vi "动力和环境监控系统状态详情.vi"() -> ()   [LabVIEW 2016, in "环境动力监测库.lvlib"]
uses:
  <vilib>/Utility/miscctls.llb/LVRowAndColumnTypeDef.ctl
  <vilib>/Utility/config.llb/NI_LVConfig.lvlib
  <vilib>/ptbypt/NI_PtbyPt.lvlib
panel:
  out "网络状态":bool
  in  "监测设备更新":bool
  in  "设备列表":i32(listbox)
  in  "add":bool
  out "设备当前时间:":timestamp format="%<%Y/%m/%d %H:%M:%S>T"
  out "当前传感器数量:":i32
  in  "设备":T1(ring)
  # "系统当前状态"
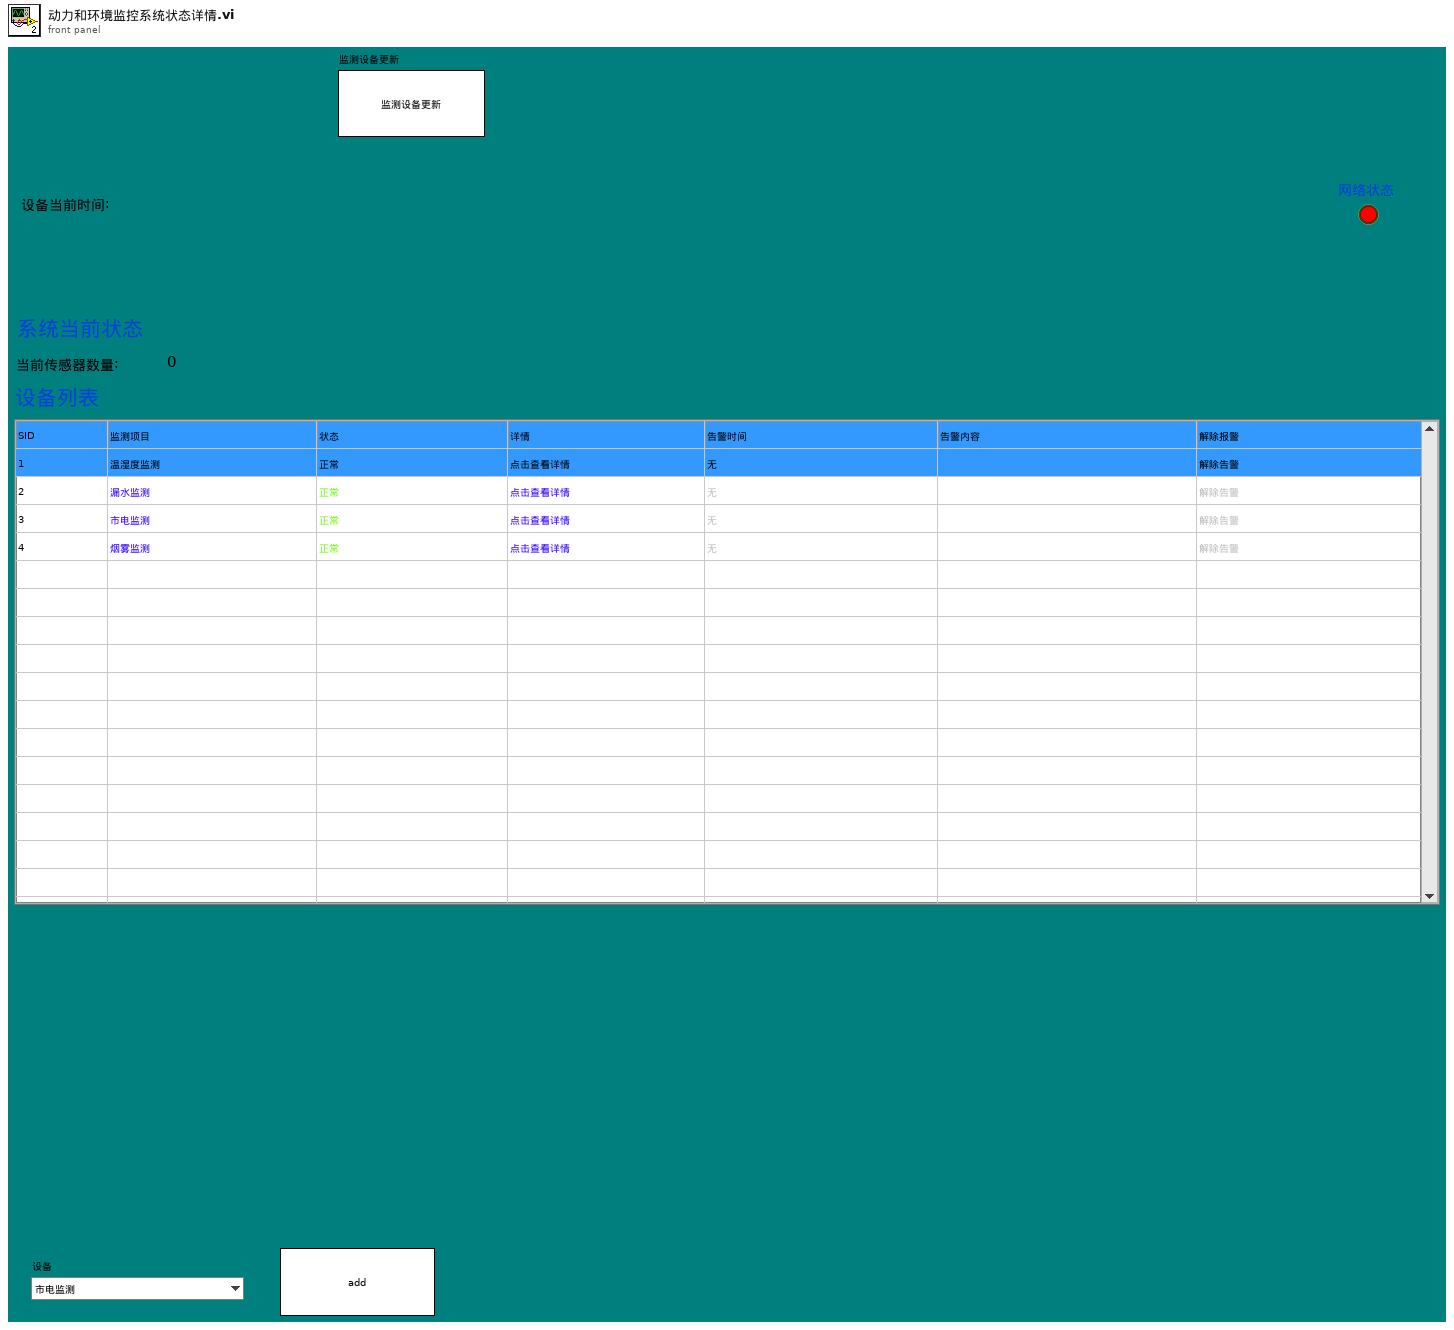
[diagram p1: front panel]
types:
  T1 = enum16{"市电监测", "UPS监测", "用水量监测", "空调监测", "烟雾监测", "温度湿度", "振动监测", "红外入侵监测", "漏水监测", "门禁开关监测", "视频监测"}
  T2 = typedef "NI_LVConfig.lvlib/Config Data RefNum.ctl" = refnum<k1>
  T3 = cluster{"市电监测":bool, "用水量监测":bool, "烟雾监测":bool, "温度湿度":bool, "振动监测":bool, "红外入侵监测":bool, "漏水监测":bool, "门禁开关监测":bool, "门禁开关监测2":bool, "视频监测":bool, "UPS监测":bool, "空调监测":bool, "冰箱监测":bool, "排气扇监测":bool, "蓄电池监测":bool, "蓄电池监测2":bool, "GPS监测":bool, "北斗监测":bool, "气象监测":bool}
  T4 = enum32{"Invalid", "Standard", "Closed", "Hidden", "Minimized", "Maximized"}
  T5 = cluster{"漏水监测输出":cluster{"漏水监测告警":bool, "告警内容":string}, "门禁监测输出":cluster{"门禁监测告警":bool, "告警内容":string}, "门禁监测输出2":cluster{"门禁监测告警":bool, "告警内容":string}, "温湿度监测输出":cluster{"温湿度监测告警":bool, "告警内容":string}, "烟雾监测输出":cluster{"烟雾监测告警":bool, "告警内容":string}, "空调监测输出":cluster{"空调监测告警":bool, "告警内容":string}, "自动重合闸输出":cluster{"自动重合闸告警":bool, "告警内容":string}, "红外入侵输出":cluster{"红外入侵告警":bool, "告警内容":string}, "振动输出":cluster{"振动告警":bool, "告警内容":string}, "UPS输出":cluster{"UPS告警":bool, "告警内容":string}, "蓄电池输出":cluster{"蓄电池告警":bool, "告警内容":string}, "蓄电池输出2":cluster{"蓄电池告警":bool, "告警内容":string}, "GPS输出":cluster{"定位告警":bool, "告警内容":string}, "北斗输出":cluster{"定位告警":bool, "告警内容":string}, "气象输出":cluster{"气象告警":bool, "告警内容":string}}
  T6 = typedef "LVRowAndColumnTypeDef.ctl" = cluster{"Row":i32, "Column":i32}
  T7 = typedef "LVPoint32TypeDef.ctl" = cluster{"Horizontal":i32, "Vertical":i32}
  T8 = enum32{"Bad", "Idle", "Run top level", "Running"}
  T9 = cluster{"AD0":dbl, "AD1":dbl, "AD1":dbl, "AD3":dbl, "AD4":dbl, "AD5":dbl, "AD6":dbl, "AD7":dbl}
  T10 = cluster{"X0":dbl, "X1":dbl, "Y0":dbl, "Y1":dbl}[]
  T11 = cluster{"AD0":dbl, "AD1":dbl, "AD2":dbl, "AD3":dbl, "AD4":dbl, "AD5":dbl, "AD6":dbl, "AD7":dbl}
  T12 = cluster{"温湿度":cluster{"状态":bool, "温度:":sgl, "湿度:":sgl, "详情  ":bool}, "空调":cluster{"状态":bool, "机柜温度:":sgl, "压缩机:":enum16{"停止", "运行"}, "电加热:":enum16{"停止", "运行"}, "详情  ":bool}, "排气扇":cluster{"排气扇:":enum16{"关闭", "打开"}, "详情  ":bool}, "冰箱":cluster{"冰箱:":enum16{"关闭", "打开"}, "详情  ":bool}}
  T13 = cluster{"市电":cluster{"状态":bool, "电压:":u16, "电流：":dbl, "详情  ":bool}, "UPS":cluster{"状态":bool, "输入电压:":sgl, "输出电压:":sgl, "电池电量:":u8, "电量":u16, "详情  ":bool}, "蓄电池12V":cluster{"状态":bool, "电压:":sgl, "电流:":sgl, "电池电量:":u8, "电量":u16, "详情  ":bool}, "蓄电池24V":cluster{"状态":bool, "电压:":sgl, "电流:":sgl, "电池电量:":u8, "电量":u16, "详情  ":bool}}
  T14 = cluster{"传感器":cluster{"红外监测":cluster{"红外监测":bool, "红外入侵监测":bool}, "振动监测":cluster{"振动监测":bool, "振动监测 2":bool}, "烟雾监测":cluster{"烟雾监测":bool, "烟雾监测 2":bool}, "门禁监测":cluster{"门禁监测":bool, "门禁开关监测":bool}, "门禁2监测":cluster{"门禁监测2":bool, "门禁开关监测2":bool}, "水浸监测":cluster{"水浸监测":bool, "漏水详情":bool}}, "气象仪":cluster{"气温: ":sgl, "气压: ":sgl, "风速:":sgl, "风向:":sgl, "气象仪经度: ":sgl, "气象仪纬度: ":sgl, "详情  ":bool}}
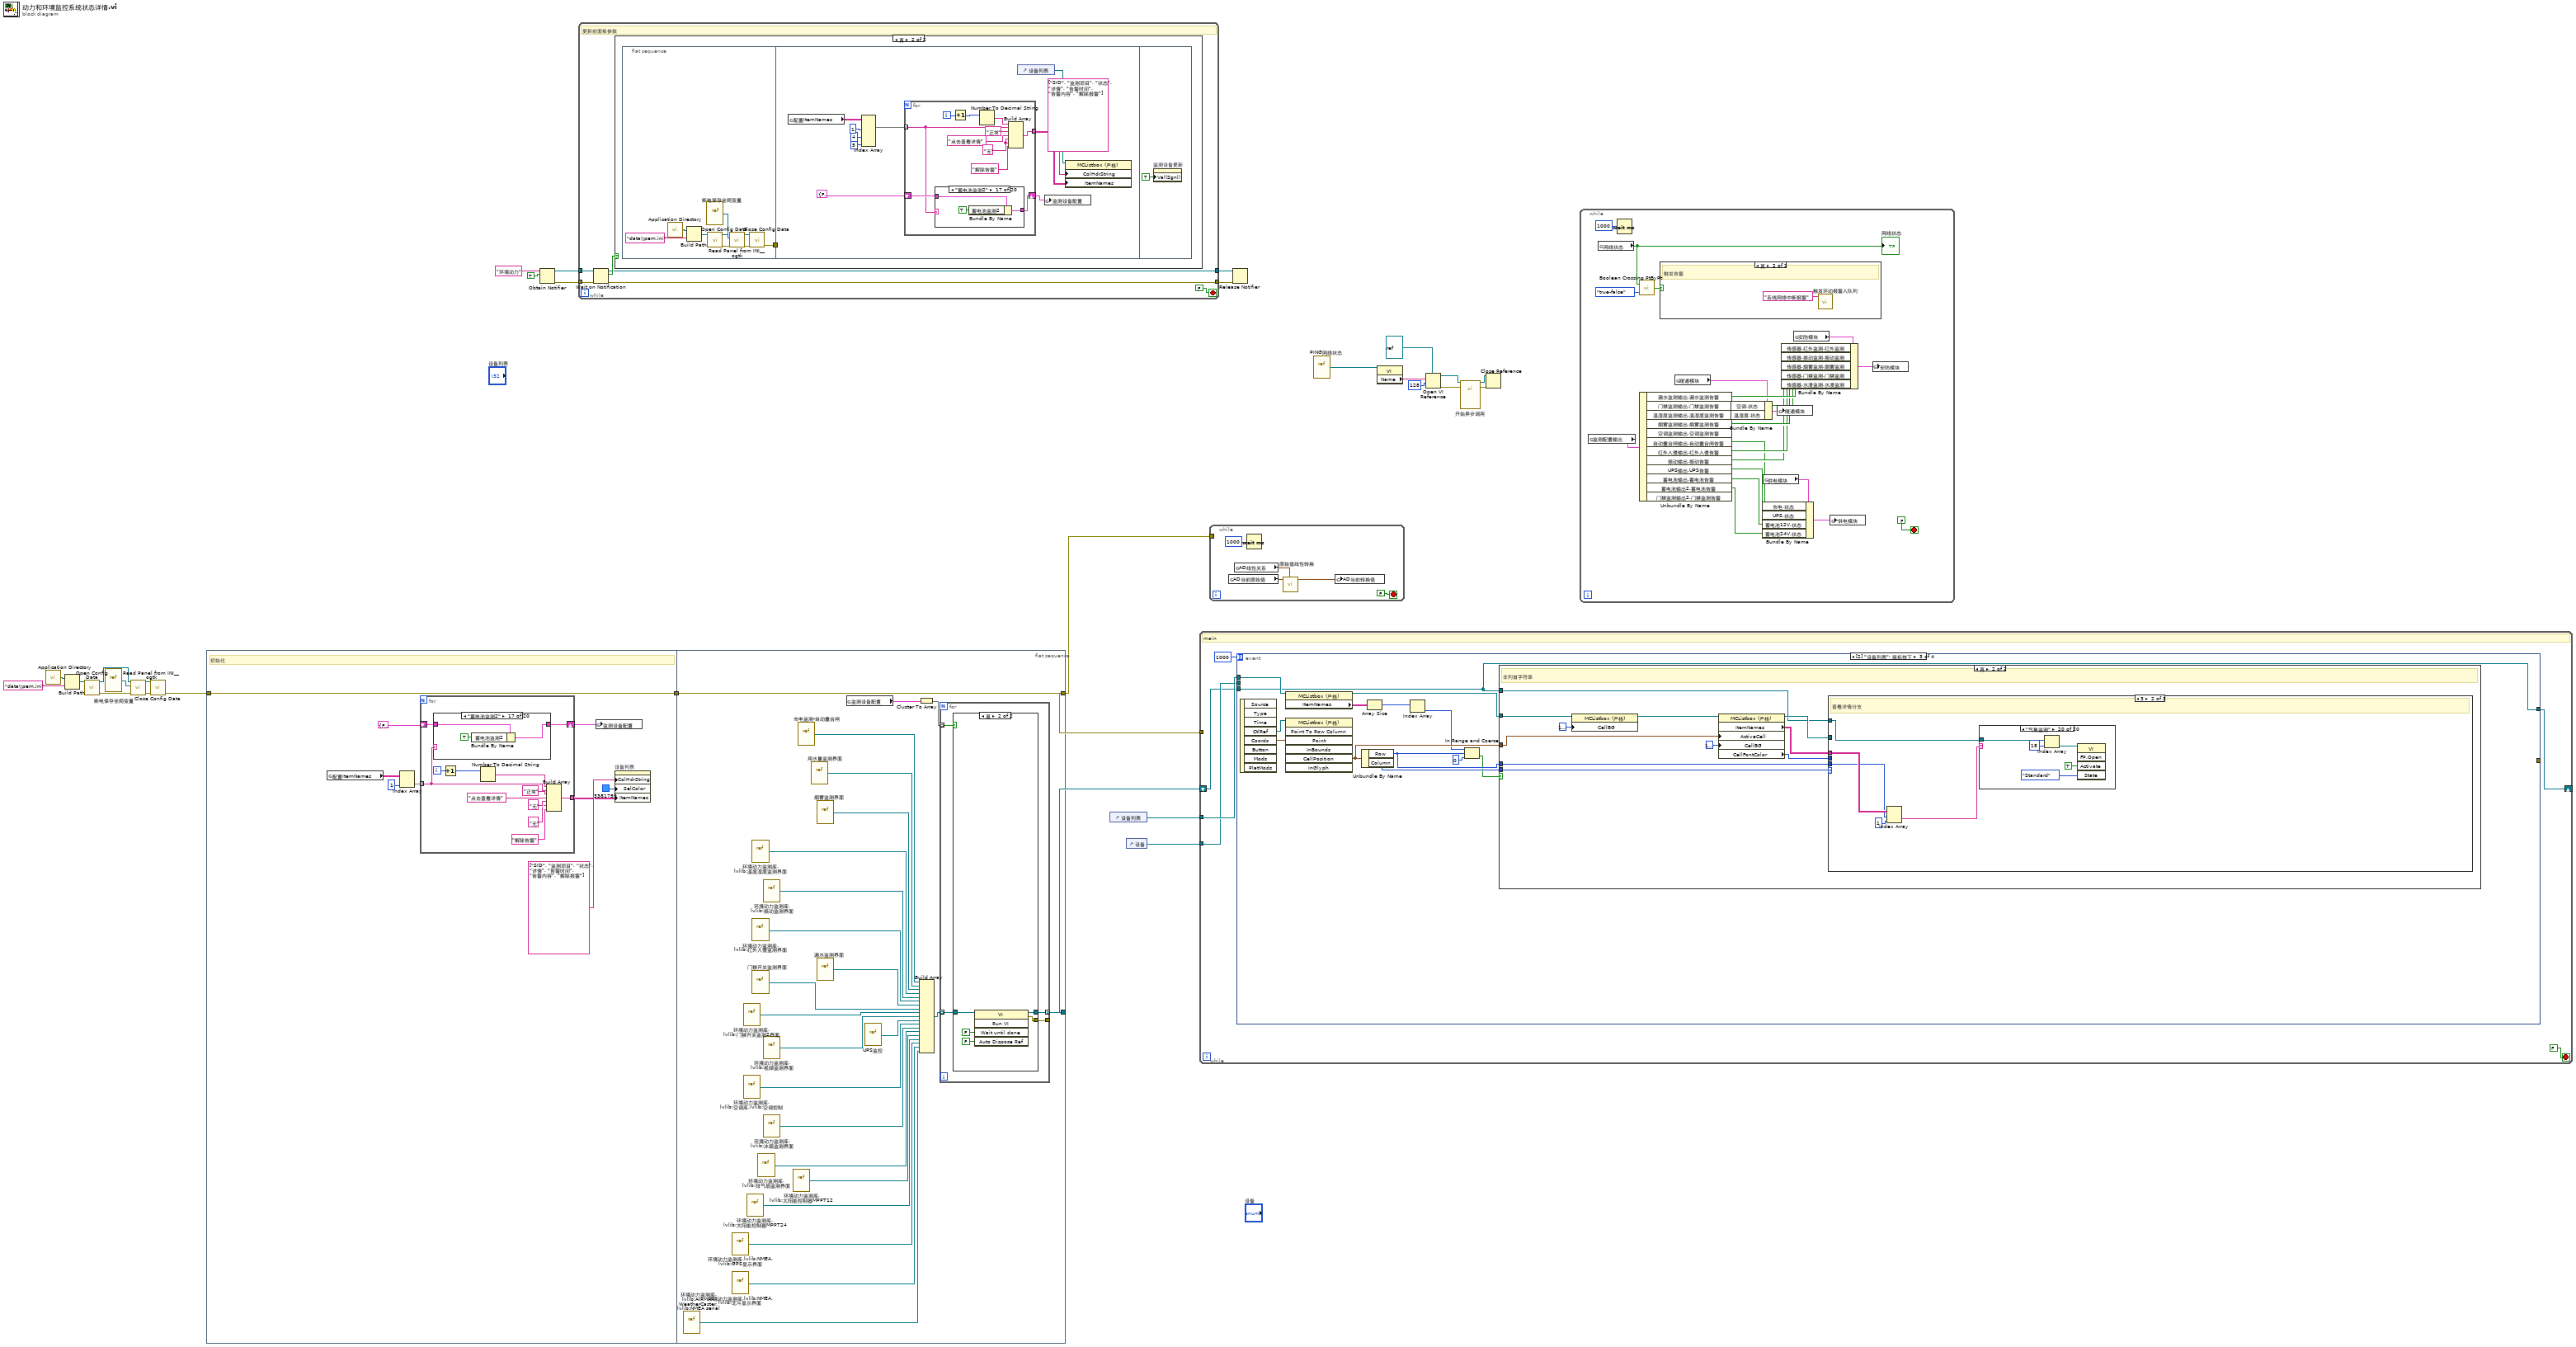
[diagram p0: block diagram]
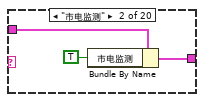
[diagram p5: hidden frame]
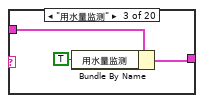
[diagram p6: hidden frame]
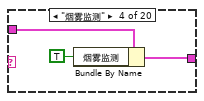
[diagram p7: hidden frame]
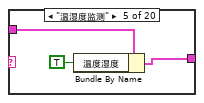
[diagram p8: hidden frame]
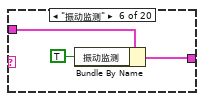
[diagram p9: hidden frame]
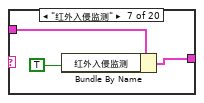
[diagram p10: hidden frame]
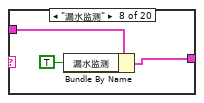
[diagram p11: hidden frame]
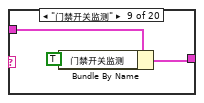
[diagram p12: hidden frame]
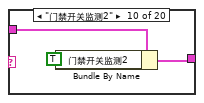
[diagram p13: hidden frame]
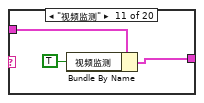
[diagram p14: hidden frame]
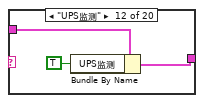
[diagram p15: hidden frame]
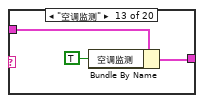
[diagram p16: hidden frame]
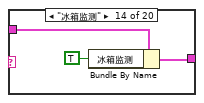
[diagram p17: hidden frame]
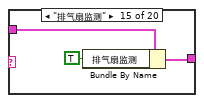
[diagram p18: hidden frame]
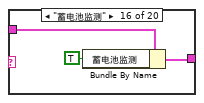
[diagram p19: hidden frame]
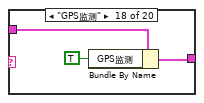
[diagram p20: hidden frame]
diagram:
  n1 = call <vilib>:"Application Directory.vi"() -> ("Application Directory"=w26:path)
  n2 = Build Path(base path=w26, name or relative path="data\\pem.ini" ("名称或相对路径")) -> (appended path=w24:path)
  n3 = call <vilib>:"Open Config Data.vi"("configuration file path"=w24) -> ("error out"=w20:errorcluster, "refnum"=w23:T2)  [unwired: 8 in, 1 out]
  n4 = vi-ref "断电保存全局变量.vi"() -> (w22:refnum<vi>)
  n5 = call <userlib>:"Read Panel from INI__ogtk.vi"("error in (no error)"=w20, "VI ref"=w22, "refnum"=w23) -> ("error out"=w19:errorcluster, "refnum out"=w21:T2)  [unwired: 7 in]
  n6 = call <vilib>:"Close Config Data.vi"("error in (no error)"=w19, "refnum"=w21) -> ("error out"=w18:errorcluster)  [unwired: 8 in, 1 out]
  n7 = flat-sequence {
    tunnel: [w31] -> w13
    tunnel: w18 -> [w31]
    tunnel: [w131] -> w1
    tunnel: w13 -> [w131]
    tunnel: [w118] -> w12
    frame #0 {
      # "初始化"
      n8 = global read "断电保存全局变量.vi" "配置ItemNames"() -> (w35:string[][])
      n9 = Index Array(array=w35, index (col)=1 ("禁用的索引 (列)")) -> (element=w33:string[])  [unwired: 1 in]
      n10 = for {
        tunnel: w33 -> [w40] mode=indexing
        tunnel: [w44] -> w32 mode=indexing
        shift-right: [w38] -> w29
        shift-left: T3 {"市电监测"=FALSE, "用水量监测"=FALSE, "烟雾监测"=FALSE, "温度湿度"=FALSE, "振动监测"=FALSE, "红外入侵监测"=FALSE, "漏水监测"=FALSE, "门禁开关监测"=FALSE, "门禁开关监测2"=FALSE, "视频监测"=FALSE, "UPS监测"=FALSE, "空调监测"=FALSE, "冰箱监测"=FALSE, "排气扇监测"=FALSE, "蓄电池监测"=FALSE, "蓄电池监测2"=FALSE, "GPS监测"=FALSE, "北斗监测"=FALSE, "气象监测"=FALSE} ("监测设备配置") -> [w39]
        i -> [w49]
        n11 = case shown="\"蓄电池监测2\"" w40 {
          tunnel: w39 -> [w50 w53 w55 w58 w61 w64 w67 w70 w73 w76 w79 w82 w85 w88 w91 w94 w97 w100 w103 w106]
          tunnel: [w50 w51 w54 w57 w60 w63 w66 w69 w72 w75 w78 w81 w84 w87 w90 w93 w96 w99 w102 w105] -> w38
          frame "假", Default {
          }
          frame "市电监测" {
            n12 = Bundle By Name(cluster=w53, "市电监测"=TRUE) -> (w51:T3)
          }
          frame "用水量监测" {
            n13 = Bundle By Name(cluster=w55, "用水量监测"=TRUE ("市电监测")) -> (w54:T3)
          }
          frame "烟雾监测" {
            n14 = Bundle By Name(cluster=w58, "烟雾监测"=TRUE ("市电监测")) -> (w57:T3)
          }
          frame "温湿度监测" {
            n15 = Bundle By Name(cluster=w61, "温度湿度"=TRUE ("市电监测")) -> (w60:T3)
          }
          frame "振动监测" {
            n16 = Bundle By Name(cluster=w64, "振动监测"=TRUE ("市电监测")) -> (w63:T3)
          }
          frame "红外入侵监测" {
            n17 = Bundle By Name(cluster=w67, "红外入侵监测"=TRUE ("市电监测")) -> (w66:T3)
          }
          frame "漏水监测" {
            n18 = Bundle By Name(cluster=w70, "漏水监测"=TRUE ("市电监测")) -> (w69:T3)
          }
          frame "门禁开关监测" {
            n19 = Bundle By Name(cluster=w73, "门禁开关监测"=TRUE ("市电监测")) -> (w72:T3)
          }
          frame "门禁开关监测2" {
            n20 = Bundle By Name(cluster=w76, "门禁开关监测2"=TRUE ("市电监测")) -> (w75:T3)
          }
          frame "视频监测" {
            n21 = Bundle By Name(cluster=w79, "视频监测"=TRUE ("市电监测")) -> (w78:T3)
          }
          frame "UPS监测" {
            n22 = Bundle By Name(cluster=w82, "UPS监测"=TRUE ("市电监测")) -> (w81:T3)
          }
          frame "空调监测" {
            n23 = Bundle By Name(cluster=w85, "空调监测"=TRUE ("市电监测")) -> (w84:T3)
          }
          frame "冰箱监测" {
            n24 = Bundle By Name(cluster=w88, "冰箱监测"=TRUE ("市电监测")) -> (w87:T3)
          }
          frame "排气扇监测" {
            n25 = Bundle By Name(cluster=w91, "排气扇监测"=TRUE ("市电监测")) -> (w90:T3)
          }
          frame "蓄电池监测" {
            n26 = Bundle By Name(cluster=w94, "蓄电池监测"=TRUE ("市电监测")) -> (w93:T3)
          }
          frame "蓄电池监测2" {
            n27 = Bundle By Name(cluster=w97, "蓄电池监测2"=TRUE ("市电监测")) -> (w96:T3)
          }
          frame "GPS监测" {
            n28 = Bundle By Name(cluster=w100, "GPS监测"=TRUE ("市电监测")) -> (w99:T3)
          }
          frame "北斗监测" {
            n29 = Bundle By Name(cluster=w103, "北斗监测"=TRUE ("市电监测")) -> (w102:T3)
          }
          frame "气象监测" {
            n30 = Bundle By Name(cluster=w106, "气象监测"=TRUE ("市电监测")) -> (w105:T3)
          }
        }
        n31 = Increment(x=w49) -> (x+1=w48:i32)
        n32 = Number To Decimal String(number=w48) -> (decimal integer string=w47:string)  [unwired: 1 in]
        n33 = Build Array(w47, w40, "正常" ("元素"), "点击查看详情" ("元素"), "无" ("元素"), "无" ("元素"), "解除告警" ("元素")) -> (w44:string[])
      }
      n34 = global write "断电保存全局变量.vi" "监测设备配置"(w29) -> ()
      n35 = property on="设备列表" class="MCListbox (严格)"("ColHdrString"=string[] ["SID", "监测项目", "状态", "详情", "告警时间", "告警内容", "解除报警"] ("列首字符串[]"), "SelColor"=u32 3381759, "ItemNames"=w32) -> ()  [unwired: 2 in, 2 out]
    }
    frame #1 {
      n36 = vi-ref "环境动力监测库.lvlib:AIRMAR WeatherCaster.lvlib:NMEA serial.vi"() -> (w114:refnum<vi>)
      n37 = vi-ref "环境动力监测库.lvlib:NMEA.lvlib:GPS显示界面.vi"() -> (w115:refnum<vi>)
      n38 = vi-ref "环境动力监测库.lvlib:NMEA.lvlib:北斗显示界面.vi"() -> (w113:refnum<vi>)
      n39 = vi-ref "环境动力监测库.lvlib:门禁开关监测2界面.vi"() -> (w109:refnum<vi>)
      n40 = vi-ref "环境动力监测库.lvlib:空调库.lvlib:空调控制.vi"() -> (w129:refnum<vi>)
      n41 = vi-ref "环境动力监测库.lvlib:太阳能控制器MPPT24.vi"() -> (w111:refnum<vi>)
      n42 = vi-ref "环境动力监测库.lvlib:温度湿度监测界面.vi"() -> (w123:refnum<vi>)
      n43 = vi-ref "环境动力监测库.lvlib:红外入侵监测界面.vi"() -> (w125:refnum<vi>)
      n44 = vi-ref "门禁开关监测界面.vi"() -> (w108:refnum<vi>)
      n45 = vi-ref "环境动力监测库.lvlib:排气扇监测界面.vi"() -> (w117:refnum<vi>)
      n46 = vi-ref "环境动力监测库.lvlib:振动监测界面.vi"() -> (w124:refnum<vi>)
      n47 = vi-ref "环境动力监测库.lvlib:视频监测界面.vi"() -> (w127:refnum<vi>)
      n48 = vi-ref "环境动力监测库.lvlib:冰箱监测界面.vi"() -> (w116:refnum<vi>)
      n49 = vi-ref "环境动力监测库.lvlib:太阳能控制器MPPT12.vi"() -> (w110:refnum<vi>)
      n50 = vi-ref "市电监测-自动重合闸.vi"() -> (w120:refnum<vi>)
      n51 = vi-ref "用水量监测界面.vi"() -> (w121:refnum<vi>)
      n52 = vi-ref "烟雾监测界面.vi"() -> (w122:refnum<vi>)
      n53 = vi-ref "漏水监测界面.vi"() -> (w126:refnum<vi>)
      n54 = global read "断电保存全局变量.vi" "监测设备配置"() -> (w112:T3)
      n55 = vi-ref "UPS监控.vi"() -> (w128:refnum<vi>)
      n56 = Cluster To Array(cluster=w112) -> (array=w130:bool[])
      n57 = Build Array(w120, w121, w122, w123, w124, w125, w126, w108, w109, w127, w128, w129, w116, w117, w110, w111, w115, w113, w114) -> (w119:refnum<vi>[])
      n58 = for {
        tunnel: w119 -> [w135] mode=indexing
        tunnel: [w134] -> w118 mode=indexing
        tunnel: w130 -> [w133] mode=indexing
        tunnel: [w132] -> _
        n59 = case shown="真" w133 {
          tunnel: w135 -> [w136 w139]
          tunnel: [w136 w138] -> w134
          tunnel: [_ w137] -> w132
          frame False {
          }
          frame True {
            n60 = invoke class="VI" method="Run VI"(reference=w139, "Wait until done"=FALSE ("结束前等待"), "Auto Dispose Ref"=FALSE ("自动销毁引用")) -> (reference out=w138:refnum<vi>, error out=w137:errorcluster)  [unwired: 2 in, 3 out]
          }
        }
      }
    }
  }
  n61 = Obtain Notifier(name (unnamed)="环境动力" ("名称（未命名）"), notification data type=TRUE) -> (notifier out=w3:refnum<notifier>, error out=w2:errorcluster)  [unwired: 2 in, 1 out]
  n62 = while {
    tunnel: w3 -> [w147]
    tunnel: w2 -> [w146]
    tunnel: [w143] -> w15
    tunnel: [w142] -> w14
    stop <- FALSE stop-if-true
    # "更新前面板参数"
    n63 = Wait on Notification(notifier=w147, error in (no error)=w146) -> (notifier out=w143:refnum<notifier>, notification=w145:bool, error out=w142:errorcluster)  [unwired: 2 in, 1 out]
    n64 = case shown="真" w145 {
      frame False {
      }
      frame True {
        n65 = flat-sequence {
          tunnel: [w149] -> w148
          tunnel: w148 -> [_]
          frame #0 {
            n66 = call <vilib>:"Application Directory.vi"() -> ("Application Directory"=w150:path)
            n67 = Build Path(base path=w150, name or relative path="data\\pem.ini" ("名称或相对路径")) -> (appended path=w152:path)
            n68 = vi-ref "断电保存全局变量.vi"() -> (w154:refnum<vi>)
            n69 = call <vilib>:"Open Config Data.vi"("configuration file path"=w152) -> ("error out"=w156:errorcluster, "refnum"=w153:T2)  [unwired: 8 in, 1 out]
            n70 = call <userlib>:"Read Panel from INI__ogtk.vi"("error in (no error)"=w156, "VI ref"=w154, "refnum"=w153) -> ("error out"=w157:errorcluster, "refnum out"=w155:T2)  [unwired: 7 in]
            n71 = call <vilib>:"Close Config Data.vi"("error in (no error)"=w157, "refnum"=w155) -> ("error out"=w149:errorcluster)  [unwired: 8 in, 1 out]
          }
          frame #1 {
            n72 = global read "断电保存全局变量.vi" "配置ItemNames"() -> (w162:string[][])
            n73 = Index Array(array=w162, index (col) #1=1 ("禁用的索引 (列)"), index (col) #2=4 ("索引 (列)"), index (col) #3=5 ("索引 (列)")) -> (element #1=w164:string[])  [unwired: 3 in, 2 out]
            n74 = for {
              tunnel: w164 -> [w170] mode=indexing
              tunnel: [w173] -> w167 mode=indexing
              shift-right: [w171] -> w161
              shift-left: T3 {"市电监测"=FALSE, "用水量监测"=FALSE, "烟雾监测"=FALSE, "温度湿度"=FALSE, "振动监测"=FALSE, "红外入侵监测"=FALSE, "漏水监测"=FALSE, "门禁开关监测"=FALSE, "门禁开关监测2"=FALSE, "视频监测"=FALSE, "UPS监测"=FALSE, "空调监测"=FALSE, "冰箱监测"=FALSE, "排气扇监测"=FALSE, "蓄电池监测"=FALSE, "蓄电池监测2"=FALSE, "GPS监测"=FALSE, "北斗监测"=FALSE, "气象监测"=FALSE} ("监测设备配置") -> [w172]
              i -> [w178]
              w168 = "无" ("元素")
              n75 = case shown="\"蓄电池监测2\"" w170 {
                tunnel: w172 -> [w179 w182 w184 w187 w190 w193 w196 w199 w202 w205 w208 w211 w214 w217 w220 w223 w226 w229 w232 w235]
                tunnel: [w179 w180 w183 w186 w189 w192 w195 w198 w201 w204 w207 w210 w213 w216 w219 w222 w225 w228 w231 w234] -> w171
                frame "假", Default {
                }
                frame "市电监测" {
                  n76 = Bundle By Name(cluster=w182, "市电监测"=TRUE) -> (w180:T3)
                }
                frame "用水量监测" {
                  n77 = Bundle By Name(cluster=w184, "用水量监测"=TRUE ("市电监测")) -> (w183:T3)
                }
                frame "烟雾监测" {
                  n78 = Bundle By Name(cluster=w187, "烟雾监测"=TRUE ("市电监测")) -> (w186:T3)
                }
                frame "温湿度监测" {
                  n79 = Bundle By Name(cluster=w190, "温度湿度"=TRUE ("市电监测")) -> (w189:T3)
                }
                frame "振动监测" {
                  n80 = Bundle By Name(cluster=w193, "振动监测"=TRUE ("市电监测")) -> (w192:T3)
                }
                frame "红外入侵监测" {
                  n81 = Bundle By Name(cluster=w196, "红外入侵监测"=TRUE ("市电监测")) -> (w195:T3)
                }
                frame "漏水监测" {
                  n82 = Bundle By Name(cluster=w199, "漏水监测"=TRUE ("市电监测")) -> (w198:T3)
                }
                frame "门禁开关监测" {
                  n83 = Bundle By Name(cluster=w202, "门禁开关监测"=TRUE ("市电监测")) -> (w201:T3)
                }
                frame "门禁开关监测2" {
                  n84 = Bundle By Name(cluster=w205, "门禁开关监测2"=TRUE ("市电监测")) -> (w204:T3)
                }
                frame "视频监测" {
                  n85 = Bundle By Name(cluster=w208, "视频监测"=TRUE ("市电监测")) -> (w207:T3)
                }
                frame "UPS监测" {
                  n86 = Bundle By Name(cluster=w211, "UPS监测"=TRUE ("市电监测")) -> (w210:T3)
                }
                frame "空调监测" {
                  n87 = Bundle By Name(cluster=w214, "空调监测"=TRUE ("市电监测")) -> (w213:T3)
                }
                frame "冰箱监测" {
                  n88 = Bundle By Name(cluster=w217, "冰箱监测"=TRUE ("市电监测")) -> (w216:T3)
                }
                frame "排气扇监测" {
                  n89 = Bundle By Name(cluster=w220, "排气扇监测"=TRUE ("市电监测")) -> (w219:T3)
                }
                frame "蓄电池监测" {
                  n90 = Bundle By Name(cluster=w223, "蓄电池监测"=TRUE ("市电监测")) -> (w222:T3)
                }
                frame "蓄电池监测2" {
                  n91 = Bundle By Name(cluster=w226, "蓄电池监测2"=TRUE ("市电监测")) -> (w225:T3)
                }
                frame "GPS监测" {
                  n92 = Bundle By Name(cluster=w229, "GPS监测"=TRUE ("市电监测")) -> (w228:T3)
                }
                frame "北斗监测" {
                  n93 = Bundle By Name(cluster=w232, "北斗监测"=TRUE ("市电监测")) -> (w231:T3)
                }
                frame "气象监测" {
                  n94 = Bundle By Name(cluster=w235, "气象监测"=TRUE ("市电监测")) -> (w234:T3)
                }
              }
              n95 = Increment(x=w178) -> (x+1=w177:i32)
              n96 = Number To Decimal String(number=w177) -> (decimal integer string=w176:string)  [unwired: 1 in]
              n97 = Build Array(w176, w170, "正常" ("元素"), "点击查看详情" ("元素"), w168, w168, "解除告警" ("元素")) -> (w173:string[])
            }
            n98 = control-ref of="设备列表"() -> (w165:refnum<vi>)
            n99 = global write "断电保存全局变量.vi" "监测设备配置"(w161) -> ()
            n100 = property class="MCListbox (严格)"(reference=w165, "ColHdrString"=string[] ["SID", "监测项目", "状态", "详情", "告警时间", "告警内容", "解除报警"] ("列首字符串[]"), "ItemNames"=w167) -> ()  [unwired: 1 in, 2 out]
          }
          frame #2 {
            n101 = property on="监测设备更新" class="Bool (严格)"("Val(Sgnl)"=TRUE ("值(信号)")) -> ()  [unwired: 2 in, 2 out]
          }
        }
      }
    }
  }
  n102 = control-ref of="设备列表"() -> (w28:refnum<vi>)
  n103 = control-ref of="设备"() -> (w27:refnum<vi>)
  n104 = while {
    tunnel: w28 -> [w242]
    tunnel: w27 -> [w241]
    tunnel: w1 -> [_]
    shift-right: [w238] -> _
    shift-left: w12 -> [w239]
    stop <- FALSE stop-if-true
    # "main"
    n105 = event shown="[2] \"设备列表\": 鼠标按下" {
      selector: _ -> [_ _ _ _]
      dyn-events: _ -> [_ _ _ _]
      timeout: 1000 -> [_ _ _ _]
      tunnel: w242 -> [_ w412 w419 _]
      tunnel: w241 -> [_ w411 _ _]
      tunnel: w239 -> [w253 w386 w413 w612]
      tunnel: [w253 w386 w413 w611] -> w238
      tunnel: [_ _ _ w595] -> _
      event Timeout {
        n106 = event-data() -> ()  [unwired: 1 in, 3 out]
        n107 = property on="设备列表" class="MCListbox (严格)"() -> (error out=w255:errorcluster, "ItemNames"=w264:string[][])  [unwired: 2 in, 1 out]
        n108 = Get Date/Time In Seconds() -> (seconds since 1Jan1904=→"设备当前时间:":timestamp)
        n109 = Array Size(array=w264) -> (size(s)=w270:i32[])
        n110 = Index Array(array=w264, index (col) #1=1 ("禁用的索引 (列)"), index (col) #2=2 ("索引 (列)"), index (col) #3=4 ("索引 (列)"), index (col) #4=5 ("索引 (列)")) -> (element #1=w262:string[], element #2=w260:string[], element #3=w247:string[], element #4=w246:string[])  [unwired: 4 in]
        n111 = global read "断电保存全局变量.vi" "监测配置输出"() -> (w252:T5)
        n112 = Index Array(array=w270) -> (element=w265:i32)  [unwired: 1 in]
        "当前传感器数量:" <- w265
        n113 = for {
          tunnel: w262 -> [w304] mode=indexing
          tunnel: w252 -> [w303]
          shift-right: [w301] -> w257
          shift-left: w260 -> [w293]
          tunnel: w255 -> [w297]
          tunnel: [w296] -> w254
          shift-right: [w292] -> w244
          shift-left: w247 -> [w287]
          shift-right: [w291] -> w245
          shift-left: w246 -> [w289]
          i -> [w277]
          w272 = u32 3342591 ("颜色盒")
          w274 = T6 {"Row"=0, "Column"=0} ("活动单元格:活动单元格")
          n114 = case shown="\"空调监测\"" w304 {
            tunnel: w303 -> [_ w325 w331 w337 w343 w349 w355 w361 w367 w372 w377 w383]
            tunnel: [FALSE ("烟雾监测输出") w321 w327 w333 w339 w345 w351 w357 w363 w369 w374 w379] -> w288
            tunnel: [_ w323 w329 w335 w341 w347 w353 w359 w365 w371 w376 w381] -> w290
            tunnel: [FALSE ("crossing") w320 w326 w332 w338 w344 w350 w356 w362 w368 w373 w378] -> w271
            frame "假", Default {
            }
            frame "市电监测" {
              n115 = Unbundle By Name(w325) -> ("自动重合闸输出"=w324:cluster{"自动重合闸告警":bool, "告警内容":string})
              n116 = Unbundle By Name(w324) -> ("自动重合闸告警"=w321:bool, "告警内容"=w323:string)
              n117 = call <vilib>:"Boolean Crossing PtByPt.vi"("direction"=enum16{"either", "false-true", "true-false"}."false-true", "input"=w321) -> ("crossing"=w320:bool)  [unwired: 1 in]
            }
            frame "空调监测" {
              n118 = Unbundle By Name(w331) -> ("空调监测输出"=w330:cluster{"空调监测告警":bool, "告警内容":string})
              n119 = Unbundle By Name(w330) -> ("空调监测告警"=w327:bool, "告警内容"=w329:string)
              n120 = call <vilib>:"Boolean Crossing PtByPt.vi"("direction"=enum16{"either", "false-true", "true-false"}."false-true", "input"=w327) -> ("crossing"=w326:bool)  [unwired: 1 in]
            }
            frame "漏水监测" {
              n121 = Unbundle By Name(w337) -> ("漏水监测输出"=w336:cluster{"漏水监测告警":bool, "告警内容":string})
              n122 = Unbundle By Name(w336) -> ("漏水监测告警"=w333:bool, "告警内容"=w335:string)
              n123 = call <vilib>:"Boolean Crossing PtByPt.vi"("direction"=enum16{"either", "false-true", "true-false"}."false-true", "input"=w333) -> ("crossing"=w332:bool)  [unwired: 1 in]
            }
            frame "门禁开关监测" {
              n124 = Unbundle By Name(w343) -> ("门禁监测输出"=w342:cluster{"门禁监测告警":bool, "告警内容":string})
              n125 = Unbundle By Name(w342) -> ("门禁监测告警"=w339:bool, "告警内容"=w341:string)
              n126 = call <vilib>:"Boolean Crossing PtByPt.vi"("direction"=enum16{"either", "false-true", "true-false"}."false-true", "input"=w339) -> ("crossing"=w338:bool)  [unwired: 1 in]
            }
            frame "温湿度监测" {
              n127 = Unbundle By Name(w349) -> ("温湿度监测输出"=w348:cluster{"温湿度监测告警":bool, "告警内容":string})
              n128 = Unbundle By Name(w348) -> ("温湿度监测告警"=w345:bool, "告警内容"=w347:string)
              n129 = call <vilib>:"Boolean Crossing PtByPt.vi"("direction"=enum16{"either", "false-true", "true-false"}."false-true", "input"=w345) -> ("crossing"=w344:bool)  [unwired: 1 in]
            }
            frame "烟雾监测" {
              n130 = Unbundle By Name(w355) -> ("烟雾监测输出"=w354:cluster{"烟雾监测告警":bool, "告警内容":string})
              n131 = Unbundle By Name(w354) -> ("烟雾监测告警"=w351:bool, "告警内容"=w353:string)
              n132 = call <vilib>:"Boolean Crossing PtByPt.vi"("direction"=enum16{"either", "false-true", "true-false"}."false-true", "input"=w351) -> ("crossing"=w350:bool)  [unwired: 1 in]
            }
            frame "UPS监测" {
              n133 = Unbundle By Name(w361) -> ("UPS输出"=w360:cluster{"UPS告警":bool, "告警内容":string})
              n134 = Unbundle By Name(w360) -> ("UPS告警"=w357:bool, "告警内容"=w359:string)
              n135 = call <vilib>:"Boolean Crossing PtByPt.vi"("direction"=enum16{"either", "false-true", "true-false"}."false-true", "input"=w357) -> ("crossing"=w356:bool)  [unwired: 1 in]
            }
            frame "蓄电池监测" {
              n136 = Unbundle By Name(w367) -> ("蓄电池输出"=w366:cluster{"蓄电池告警":bool, "告警内容":string})
              n137 = Unbundle By Name(w366) -> ("蓄电池告警"=w363:bool, "告警内容"=w365:string)
              n138 = call <vilib>:"Boolean Crossing PtByPt.vi"("direction"=enum16{"either", "false-true", "true-false"}."false-true", "input"=w363) -> ("crossing"=w362:bool)  [unwired: 1 in]
            }
            frame "GPS监测" {
              n139 = Unbundle By Name(w372) -> ("GPS输出.定位告警"=w369:bool, "GPS输出.告警内容"=w371:string)
              n140 = call <vilib>:"Boolean Crossing PtByPt.vi"("direction"=enum16{"either", "false-true", "true-false"}."false-true", "input"=w369) -> ("crossing"=w368:bool)  [unwired: 1 in]
            }
            frame "北斗监测" {
              n141 = Unbundle By Name(w377) -> ("北斗输出.定位告警"=w374:bool, "北斗输出.告警内容"=w376:string)
              n142 = call <vilib>:"Boolean Crossing PtByPt.vi"("direction"=enum16{"either", "false-true", "true-false"}."false-true", "input"=w374) -> ("crossing"=w373:bool)  [unwired: 1 in]
            }
            frame "气象监测" {
              n143 = Unbundle By Name(w383) -> ("气象输出"=w382:cluster{"气象告警":bool, "告警内容":string})
              n144 = Unbundle By Name(w382) -> ("气象告警"=w379:bool, "告警内容"=w381:string)
              n145 = call <vilib>:"Boolean Crossing PtByPt.vi"("direction"=enum16{"either", "false-true", "true-false"}."false-true", "input"=w379) -> ("crossing"=w378:bool)  [unwired: 1 in]
            }
          }
          n146 = case shown="真" w288 {
            tunnel: ["正常" "报警"] -> w302
            tunnel: [u32 6618880 u32 16711680] -> w298
            tunnel: [u32 12369084 u32 3342591 ("颜色盒")] -> w280
            frame False {
            }
            frame True {
            }
          }
          n147 = Index Array(array=w287, index=w277) -> (element=w286:string)
          n148 = Replace Array Subset(array=w289, new element=w290, index=w277) -> (w291:string[])
          n149 = case shown="假" w271 {
            tunnel: [w305 w306] -> w285
            tunnel: w286 -> [w305 _]
            frame False {
            }
            frame True {
              n150 = Get Date/Time In Seconds() -> (seconds since 1Jan1904=w311:timestamp)
              n151 = Get Date/Time String(date format (0)=enum16{"short", "long", "abbreviated"}."long" ("日期格式(0)"), seconds (now)=w311, want seconds? (F)=TRUE ("需要秒？(F)")) -> (date string=w308:string, time string=w307:string)
              n152 = Concatenate Strings(w308, w307) -> (w306:string)
            }
          }
          n153 = Bundle By Name(cluster=w274, "Row"=w277, "Column"=4) -> (w282:T6)
          n154 = Bundle By Name(cluster=w274, "Row"=w277, "Column"=2) -> (w299:T6)
          n155 = Bundle By Name(cluster=w274, "Row"=w277, "Column"=6) -> (w294:T6)
          n156 = Bundle By Name(cluster=w274, "Row"=w277, "Column"=5) -> (w281:T6)
          n157 = Bundle By Name(cluster=w274, "Row"=w277, "Column"=1) -> (w276:T6)
          n158 = Bundle By Name(cluster=w274, "Row"=w277, "Column"=3) -> (w273:T6)
          n159 = property on="设备列表" class="MCListbox (严格)"(error in=w297, "ActiveCell"=w299, "CellFontColor"=w298, "ActiveCell"=w294, "CellFontColor"=w280, "ActiveCell"=w282, "CellFontColor"=w280, "ActiveCell"=w281, "CellFontColor"=w280, "ActiveCell"=w276, "CellFontBold"=TRUE ("活动单元格:单元格字体:粗体"), "CellFontColor"=w272, "ActiveCell"=w273, "CellFontColor"=w272) -> (error out=w296:errorcluster)  [unwired: 1 in, 1 out]
          n160 = Replace Array Subset(array=w293, new element=w302, index=w277) -> (w301:string[])
          n161 = Replace Array Subset(array=w287, new element=w285, index=w277) -> (w292:string[])
        }
        n162 = for {
          N: w265 -> [_]
          tunnel: [w384] -> w269 mode=indexing
          i -> [w385]
          n163 = Increment(x=w385) -> (x+1=w384:i32)
        }
        n164 = Number To Decimal String(number=w269) -> (decimal integer string=w268:string[])  [unwired: 1 in]
        n165 = Replace Array Subset(array=w264, new element=w268, index (col)=0 ("禁用的索引 (列)")) -> (w259:string[][])  [unwired: 1 in]
        n166 = Replace Array Subset(array=w259, new element #1=w257, index (col) #1=2 ("禁用的索引 (列)"), new element #2=w244, index (col) #2=4 ("索引 (列)"), new element #3=w245, index (col) #3=5 ("索引 (列)")) -> (w256:string[][])  [unwired: 3 in]
        n167 = property on="设备列表" class="MCListbox (严格)"(error in=w254, "ItemNames"=w256) -> ()  [unwired: 1 in, 2 out]
      }
      event "add": Value Change {
        w388 = u32 3342591 ("颜色盒")
        n168 = event-data() -> ()  [unwired: 1 in, 6 out]
        n169 = property class="MCListbox (严格)"(reference=w412) -> (reference out=w401:refnum<vi>, "ItemNames"=w405:string[][])  [unwired: 1 in, 1 out]
        n170 = property class="Enum (严格)"(reference=w411) -> ("RingText.Text"=w410:string)  [unwired: 1 in, 2 out]
        n171 = Array Size(array=w405) -> (size(s)=w404:i32[])
        n172 = Index Array(array=w404) -> (element=w393:i32)  [unwired: 1 in]
        n173 = Increment(x=w393) -> (x+1=w403:i32)
        n174 = Number To Decimal String(number=w403) -> (decimal integer string=w402:string)  [unwired: 1 in]
        n175 = Build Array(w402, w410, "正常" ("元素"), "点击查看详情" ("元素"), "解除告警" ("元素")) -> (w409:string[])
        n176 = Build Array (concatenate)(w405, w409) -> (w390:string[][])
        n177 = Bundle(w393, "Column"=1) -> (w389:cluster{i32, "Column":i32})  [unwired: 1 in]
        n178 = Bundle(w393, "Column"=2) -> (w398:cluster{i32, "Column":i32})  [unwired: 1 in]
        n179 = Bundle(w393, "Column"=3) -> (w395:cluster{i32, "Column":i32})  [unwired: 1 in]
        n180 = Bundle(w393, "Column"=4) -> (w392:cluster{i32, "Column":i32})  [unwired: 1 in]
        n181 = property class="MCListbox (严格)"(reference=w401, "ItemNames"=w390, "ActiveCell"=w389, "CellFontColor"=w388, "CellFontBold"=TRUE ("活动单元格:单元格字体:斜体"), "ActiveCell"=w398, "CellFontColor"=u32 61277 ("颜色盒"), "ActiveCell"=w395, "CellFontColor"=w388, "ActiveCell"=w392, "CellFontColor"=u32 12369084 ("颜色盒")) -> ()  [unwired: 1 in, 2 out]
      }
      event "设备列表": Mouse Down {
        n182 = event-data() -> ("CtlRef"=w425:refnum<vi>, "Coords"=w423:T7)  [unwired: 1 in, 6 out]
        n183 = property class="MCListbox (严格)"(reference=w419) -> (reference out=w415:refnum<vi>, "ItemNames"=w418:string[][])  [unwired: 1 in, 1 out]
        n184 = invoke class="MCListbox (严格)" method="Point To Row Column"(reference=w425, "Point"=w423) -> ("CellPosition"=w422:T6)  [unwired: 5 in, 6 out]
        n185 = Unbundle By Name(w422) -> ("Row"=w421:i32, "Column"=w424:i32)
        n186 = Array Size(array=w418) -> (size(s)=w417:i32[])
        n187 = Index Array(array=w417) -> (element=w416:i32)  [unwired: 1 in]
        n188 = In Range and Coerce(upper limit=w416, x=w421, lower limit=0 ("下限")) -> (In Range?=w414:bool)  [unwired: 1 out]
        n189 = case shown="真" w414 {
          tunnel: w424 -> [_ w435]
          tunnel: w421 -> [_ w434]
          tunnel: w422 -> [_ w432]
          tunnel: w415 -> [_ w429]
          tunnel: w413 -> [_ w426]
          frame False {
          }
          frame True {
            # "非列首字符串"
            n190 = property class="MCListbox (严格)"(reference=w429, "CellBG"=u32 16777216) -> (reference out=w430:refnum<vi>)  [unwired: 1 in, 1 out]
            n191 = property class="MCListbox (严格)"(reference=w430, "ActiveCell"=w432, "CellBG"=u32 16777216) -> (reference out=w433:refnum<vi>, "ItemNames"=w436:string[][], "CellFontColor"=w427:u32)  [unwired: 1 in, 1 out]
            n192 = case shown="3" w435 {
              tunnel: w436 -> [_ w441 w544]
              tunnel: w434 -> [_ w439 w542]
              tunnel: w433 -> [_ _ w543]
              tunnel: w427 -> [_ _ w541]
              tunnel: w426 -> [_ w437 _]
              frame 0, Default {
              }
              frame 3 {
                # "查看详情分支"
                n193 = Index Array(array=w441, index (row)=w439, index (col)=1 ("禁用的索引 (列)")) -> (element=w438:string)
                n194 = case shown="\"气象监测\"" w438 {
                  selector: w438 -> [w442 _ _ _ _ _ _ _ _ _ _ _ _ _ _ _ _ _ _ _]
                  tunnel: w437 -> [_ w446 w451 w456 w461 w466 w471 w476 w481 w486 w490 w495 w500 w505 w510 w515 w520 w525 w530 w535]
                  frame "假", Default {
                    n195 = Concatenate Strings(w442, "详情" ("字符串")) -> (w444:string)
                    n196 = One Button Dialog(message=w444) -> ()  [unwired: 1 in, 1 out]
                  }
                  frame "市电监测" {
                    n197 = Index Array(array=w446) -> (element=w445:refnum<vi>)  [unwired: 1 in]
                    n198 = invoke class="VI" method="FP.Open"(reference=w445, "Activate"=TRUE ("激活？"), "State"=T4."Standard" ("状态")) -> ()  [unwired: 2 in, 5 out]
                  }
                  frame "用水量监测" {
                    n199 = Index Array(array=w451, index=1 ("索引")) -> (element=w449:refnum<vi>)
                    n200 = invoke class="VI" method="FP.Open"(reference=w449, "Activate"=TRUE ("激活？"), "State"=T4."Standard" ("状态")) -> ()  [unwired: 2 in, 5 out]
                  }
                  frame "烟雾监测" {
                    n201 = Index Array(array=w456, index=2 ("索引")) -> (element=w454:refnum<vi>)
                    n202 = invoke class="VI" method="FP.Open"(reference=w454, "Activate"=TRUE ("激活？"), "State"=T4."Standard" ("状态")) -> ()  [unwired: 2 in, 5 out]
                  }
                  frame "温湿度监测" {
                    n203 = Index Array(array=w461, index=3 ("索引")) -> (element=w459:refnum<vi>)
                    n204 = invoke class="VI" method="FP.Open"(reference=w459, "Activate"=TRUE ("激活？"), "State"=T4."Standard" ("状态")) -> ()  [unwired: 2 in, 5 out]
                  }
                  frame "振动监测" {
                    n205 = Index Array(array=w466, index=4 ("索引")) -> (element=w464:refnum<vi>)
                    n206 = invoke class="VI" method="FP.Open"(reference=w464, "Activate"=TRUE ("激活？"), "State"=T4."Standard" ("状态")) -> ()  [unwired: 2 in, 5 out]
                  }
                  frame "红外入侵监测" {
                    n207 = Index Array(array=w471, index=5 ("索引")) -> (element=w469:refnum<vi>)
                    n208 = invoke class="VI" method="FP.Open"(reference=w469, "Activate"=TRUE ("激活？"), "State"=T4."Standard" ("状态")) -> ()  [unwired: 2 in, 5 out]
                  }
                  frame "漏水监测" {
                    n209 = Index Array(array=w476, index=6 ("索引")) -> (element=w474:refnum<vi>)
                    n210 = invoke class="VI" method="FP.Open"(reference=w474, "Activate"=TRUE ("激活？"), "State"=T4."Standard" ("状态")) -> ()  [unwired: 2 in, 5 out]
                  }
                  frame "门禁开关监测" {
                    n211 = Index Array(array=w481, index=7 ("索引")) -> (element=w479:refnum<vi>)
                    n212 = invoke class="VI" method="FP.Open"(reference=w479, "Activate"=TRUE ("激活？"), "State"=T4."Standard" ("状态")) -> ()  [unwired: 2 in, 5 out]
                  }
                  frame "门禁开关监测2" {
                    n213 = Index Array(array=w486, index=8 ("索引")) -> (element=w484:refnum<vi>)
                    n214 = invoke class="VI" method="FP.Open"(reference=w484, "Activate"=TRUE ("激活？"), "State"=T4."Standard" ("状态")) -> ()  [unwired: 2 in, 5 out]
                  }
                  frame "视频监测" {
                    n215 = Index Array(array=w490, index=9 ("索引")) -> (element=w489:refnum<vi>)
                    n216 = invoke class="VI" method="FP.Open"(reference=w489, "Activate"=TRUE ("激活？"), "State"=T4."Standard" ("状态")) -> ()  [unwired: 2 in, 5 out]
                  }
                  frame "UPS监测" {
                    n217 = Index Array(array=w495, index=10 ("索引")) -> (element=w494:refnum<vi>)
                    n218 = invoke class="VI" method="FP.Open"(reference=w494, "Activate"=TRUE ("激活？"), "State"=T4."Standard" ("状态")) -> ()  [unwired: 2 in, 5 out]
                  }
                  frame "空调监测" {
                    n219 = Index Array(array=w500, index=11 ("索引")) -> (element=w499:refnum<vi>)
                    n220 = invoke class="VI" method="FP.Open"(reference=w499, "Activate"=TRUE ("激活？"), "State"=T4."Standard" ("状态")) -> ()  [unwired: 2 in, 5 out]
                  }
                  frame "冰箱监测" {
                    n221 = Index Array(array=w505, index=12 ("索引")) -> (element=w504:refnum<vi>)
                    n222 = invoke class="VI" method="FP.Open"(reference=w504, "Activate"=TRUE ("激活？"), "State"=T4."Standard" ("状态")) -> ()  [unwired: 2 in, 5 out]
                  }
                  frame "排气扇监测" {
                    n223 = Index Array(array=w510, index=13 ("索引")) -> (element=w509:refnum<vi>)
                    n224 = invoke class="VI" method="FP.Open"(reference=w509, "Activate"=TRUE ("激活？"), "State"=T4."Standard" ("状态")) -> ()  [unwired: 2 in, 5 out]
                  }
                  frame "蓄电池监测" {
                    n225 = Index Array(array=w515, index=14 ("索引")) -> (element=w514:refnum<vi>)
                    n226 = invoke class="VI" method="FP.Open"(reference=w514, "Activate"=TRUE ("激活？"), "State"=T4."Standard" ("状态")) -> ()  [unwired: 2 in, 5 out]
                  }
                  frame "蓄电池监测2" {
                    n227 = Index Array(array=w520, index=15 ("索引")) -> (element=w519:refnum<vi>)
                    n228 = invoke class="VI" method="FP.Open"(reference=w519, "Activate"=TRUE ("激活？"), "State"=T4."Standard" ("状态")) -> ()  [unwired: 2 in, 5 out]
                  }
                  frame "GPS监测" {
                    n229 = Index Array(array=w525, index=16 ("索引")) -> (element=w524:refnum<vi>)
                    n230 = invoke class="VI" method="FP.Open"(reference=w524, "Activate"=TRUE ("激活？"), "State"=T4."Standard" ("状态")) -> ()  [unwired: 2 in, 5 out]
                  }
                  frame "北斗监测" {
                    n231 = Index Array(array=w530, index=17 ("索引")) -> (element=w529:refnum<vi>)
                    n232 = invoke class="VI" method="FP.Open"(reference=w529, "Activate"=TRUE ("激活？"), "State"=T4."Standard" ("状态")) -> ()  [unwired: 2 in, 5 out]
                  }
                  frame "气象监测" {
                    n233 = Index Array(array=w535, index=18 ("索引")) -> (element=w534:refnum<vi>)
                    n234 = invoke class="VI" method="FP.Open"(reference=w534, "Activate"=TRUE ("激活？"), "State"=T4."Standard" ("状态")) -> ()  [unwired: 2 in, 5 out]
                  }
                }
              }
              frame 6 {
                # "解除报警"
                n235 = Equal?(x=w541, y=u32 3342591 ("颜色盒")) -> (x = y?=w540:bool)
                n236 = case shown="真" w540 {
                  tunnel: w544 -> [_ w549]
                  tunnel: w543 -> [_ _]
                  tunnel: w542 -> [_ w548]
                  frame False {
                  }
                  frame True {
                    n237 = Index Array(array=w549, index (row)=w548, index (col)=1 ("禁用的索引 (列)")) -> (element=w545:string)
                    n238 = Format Into String(format string="是否解除%s报警？" ("消息"), w545) -> (resulting string=w550:string)  [unwired: 2 in, 1 out]
                    n239 = Two Button Dialog(message=w550) -> (T button?=w546:bool)  [unwired: 2 in]
                    n240 = case shown="真" w546 {
                      tunnel: w545 -> [_ w552]
                      frame False {
                      }
                      frame True {
                        # "触发解除报警事件"
                        n241 = global read "断电保存全局变量.vi" "监测配置输出"() -> (w553:T5)
                        n242 = case shown="\"蓄电池监测2\"" w552 {
                          tunnel: w553 -> [w556 w559 w562 w565 w568 w570 w574 w577 w579 w582 w585 w588 w591]
                          tunnel: [w556 w558 w561 w564 w567 w569 w572 w576 w578 w581 w584 w587 w590] -> w554
                          tunnel: FALSE ("烟雾监测输出") -> [_ w557 w560 w563 w566 w571 w573 w575 w580 w583 w586 w589 w592]
                          frame "假", Default {
                          }
                          frame "市电监测" {
                            n243 = Bundle By Name(cluster=w559, "自动重合闸输出.自动重合闸告警"=w557) -> (w558:T5)
                          }
                          frame "空调监测" {
                            n244 = Bundle By Name(cluster=w562, "空调监测输出.空调监测告警"=w560) -> (w561:T5)
                          }
                          frame "漏水监测" {
                            n245 = Bundle By Name(cluster=w565, "漏水监测输出.漏水监测告警"=w563) -> (w564:T5)
                          }
                          frame "门禁开关监测" {
                            n246 = Bundle By Name(cluster=w568, "门禁监测输出.门禁监测告警"=w566) -> (w567:T5)
                          }
                          frame "温湿度监测" {
                            n247 = Bundle By Name(cluster=w570, "温湿度监测输出.温湿度监测告警"=w571) -> (w569:T5)
                          }
                          frame "烟雾监测" {
                            n248 = Bundle By Name(cluster=w574, "烟雾监测输出.烟雾监测告警"=w573) -> (w572:T5)
                          }
                          frame "UPS监测" {
                            n249 = Bundle By Name(cluster=w577, "UPS输出.UPS告警"=w575) -> (w576:T5)
                          }
                          frame "蓄电池监测" {
                            n250 = Bundle By Name(cluster=w579, "蓄电池输出.蓄电池告警"=w580) -> (w578:T5)
                          }
                          frame "蓄电池监测2" {
                            n251 = Bundle By Name(cluster=w582, "蓄电池输出2.蓄电池告警"=w583) -> (w581:T5)
                          }
                          frame "GPS监测" {
                            n252 = Bundle By Name(cluster=w585, "GPS输出.定位告警"=w586) -> (w584:T5)
                          }
                          frame "北斗监测" {
                            n253 = Bundle By Name(cluster=w588, "北斗输出.定位告警"=w589) -> (w587:T5)
                          }
                          frame "气象监测" {
                            n254 = Bundle By Name(cluster=w591, "气象输出.气象告警"=w592) -> (w590:T5)
                          }
                        }
                        n255 = global write "断电保存全局变量.vi" "监测配置输出"(w554) -> ()
                      }
                    }
                  }
                }
              }
            }
          }
        }
      }
      event "监测设备更新": Value Change {
        n256 = event-data() -> ()  [unwired: 1 in, 6 out]
        n257 = global read "断电保存全局变量.vi" "监测设备配置"() -> (w610:T3)
        n258 = Cluster To Array(cluster=w610) -> (array=w613:bool[])
        n259 = for {
          tunnel: w612 -> [w617] mode=indexing
          tunnel: [w616] -> w611 mode=indexing
          tunnel: w613 -> [w615] mode=indexing
          tunnel: [w614] -> w594
          n260 = case shown="假" w615 {
            tunnel: w617 -> [w620 w623]
            tunnel: [w619 w625] -> w616
            tunnel: [w618 w624] -> w614
            frame False {
              n261 = invoke class="VI" method="Abort VI"(reference=w620) -> (reference out=w619:refnum<vi>, error out=w618:errorcluster)  [unwired: 2 in, 1 out]
            }
            frame True {
              n262 = property class="VI"(reference=w623) -> (reference out=w621:refnum<vi>, "Exec.State"=w622:T8)  [unwired: 1 in, 1 out]
              n263 = case shown="\"Idle\"" w622 {
                tunnel: [w626 w629] -> w625
                tunnel: [_ w628] -> w624
                tunnel: w621 -> [w626 w627]
                frame "Bad", Default {
                }
                frame "Idle" {
                  n264 = invoke class="VI" method="Run VI"(reference=w627, "Wait until done"=FALSE ("结束前等待"), "Auto Dispose Ref"=FALSE ("自动销毁引用")) -> (reference out=w629:refnum<vi>, error out=w628:errorcluster)  [unwired: 2 in, 3 out]
                }
              }
            }
          }
        }
        n265 = call <vilib>:"Clear Errors.vi"("error in (no error)"=w594) -> ("error out"=w593:errorcluster)  [unwired: 5 in, 1 out]
        n266 = call <vilib>:"Application Directory.vi"() -> ("Application Directory"=w609:path)
        n267 = Build Path(base path=w609, name or relative path="data\\pem.ini" ("名称或相对路径")) -> (appended path=w607:path)
        n268 = call <vilib>:"Open Config Data.vi"("error in (no error)"=w593, "configuration file path"=w607) -> ("error out"=w605:errorcluster, "refnum"=w606:T2)  [unwired: 7 in, 1 out]
        n269 = vi-ref "断电保存全局变量.vi"() -> (w596:refnum<vi>)
        n270 = call <userlib>:"Write Panel to INI__ogtk.vi"("error in (no error)"=w605, "VI ref"=w596, "refnum"=w606) -> ("error out"=w603:errorcluster, "refnum out"=w604:T2)  [unwired: 7 in]
        n271 = call <vilib>:"Close Config Data.vi"("error in (no error)"=w603, "refnum"=w604) -> ("error out"=w597:errorcluster, "file path"=w598:path)  [unwired: 8 in]
        n272 = Open/Create/Replace File(file path (use dialog)=w598, error in=w597) -> (refnum out=w601:refnum<file>, error out=w602:errorcluster)  [unwired: 4 in, 1 out]
        n273 = Flush File(refnum=w601, error in=w602) -> (refnum out=w600:refnum<file>, error out=w599:errorcluster)
        n274 = Close File(refnum=w600, error in=w599) -> (error out=w595:errorcluster)  [unwired: 1 out]
      }
    }
  }
  n275 = while {
    tunnel: w1 -> [_]
    stop <- FALSE stop-if-true
    n276 = global read "断电保存全局变量.vi" "AD当前原始值"() -> (w634:T9)
    n277 = global read "断电保存全局变量.vi" "AD线性关系"() -> (w632:T10)
    n278 = Wait (ms)(milliseconds to wait=u32 1000 ("等待时间（毫秒）")) -> ()  [unwired: 1 out]
    n279 = call "原始值线性转换.vi"("AD线性关系"=w632, "AD当前原始值"=w634) -> ("AD当前转换值"=w633:T11)  [unwired: 9 in]
    n280 = global write "断电保存全局变量.vi" "AD当前转换值"(w633) -> ()
  }
  n281 = Release Notifier(notifier=w15, error in (no error)=w14) -> ()  [unwired: 1 in, 3 out]
  n282 = vi-ref "PING网络状态.vi"() -> (w4:refnum<vi>)
  n283 = property class="VI"(reference=w4) -> ("Name"=w11:string)  [unwired: 1 in, 2 out]
  n284 = Open VI Reference(type specifier VI Refnum (for type only)=refnum<vi> refnum, vi path=w11, options=128 ("选项")) -> (vi reference=w9:refnum<vi>, error out=w7:errorcluster)  [unwired: 3 in]
  n285 = call-by-ref "开始异步调用"(reference=w9, error in=w7) -> (reference out=w5:refnum<vi>, error out=w6:errorcluster)  [unwired: 12 in]
  n286 = Close Reference(reference=w5, error in (no error)=w6) -> ()  [unwired: 1 out]
  n287 = while {
    stop <- FALSE stop-if-true
    n288 = global read "断电保存全局变量.vi" "监测配置输出"() -> (w652:T5)
    n289 = global read "内部交互全局变量.vi" "网络状态"() -> (w655:bool)
    "网络状态" <- w655
    n290 = Wait (ms)(milliseconds to wait=u32 1000 ("等待时间（毫秒）")) -> ()  [unwired: 1 out]
    n291 = Unbundle By Name(w652) -> ("漏水监测输出.漏水监测告警"=w651:bool, "门禁监测输出.门禁监测告警"=w650:bool, "温湿度监测输出.温湿度监测告警"=w638:bool, "烟雾监测输出.烟雾监测告警"=w649:bool, "空调监测输出.空调监测告警"=w639:bool, "自动重合闸输出.自动重合闸告警"=w644:bool, "红外入侵输出.红外入侵告警"=w648:bool, "振动输出.振动告警"=w647:bool, "UPS输出.UPS告警"=w643:bool, "蓄电池输出.蓄电池告警"=w642:bool, "蓄电池输出2.蓄电池告警"=w637:bool)  [unwired: 1 out]
    n292 = call <vilib>:"Boolean Crossing PtByPt.vi"("direction"=enum16{"either", "false-true", "true-false"}."true-false", "input"=w655) -> ("crossing"=w656:bool)  [unwired: 1 in]
    n293 = case shown="真" w656 {
      frame False {
      }
      frame True {
        # "触发告警"
        n294 = call "触发环动报警入队列.vi"("报警内容"="系统网络中断报警") -> ()  [unwired: 11 in]
      }
    }
    n295 = global read "内部交互全局变量.vi" "暖通模块"() -> (w641:T12)
    n296 = Bundle By Name(cluster=w641, "空调.状态"=w639, "温湿度.状态"=w638) -> (w640:T12)
    n297 = global read "内部交互全局变量.vi" "供电模块"() -> (w645:T13)
    n298 = Bundle By Name(cluster=w645, "市电.状态"=w644, "UPS.状态"=w643, "蓄电池12V.状态"=w642, "蓄电池24V.状态"=w637) -> (w646:T13)
    n299 = global write "内部交互全局变量.vi" "暖通模块"(w640) -> ()
    n300 = global read "内部交互全局变量.vi" "安防模块"() -> (w654:T14)
    n301 = Bundle By Name(cluster=w654, "传感器.红外监测.红外监测"=w648, "传感器.振动监测.振动监测"=w647, "传感器.烟雾监测.烟雾监测"=w649, "传感器.门禁监测.门禁监测"=w650, "传感器.水浸监测.水浸监测"=w651) -> (w653:T14)
    n302 = global write "内部交互全局变量.vi" "供电模块"(w646) -> ()
    n303 = global write "内部交互全局变量.vi" "安防模块"(w653) -> ()
  }
